vi "Scale Spectrum Information.vi"(8 "error in (no error)":errorcluster, 11 "Spectral Information (DBFS)":dbl[](array[numeric])) -> (0 "error out":errorcluster, 3 "Spectral Waveform":waveform(dbl))   [LabVIEW 2016]
uses:
  RTLSDR Control/RTLSDR Global Variables.vi
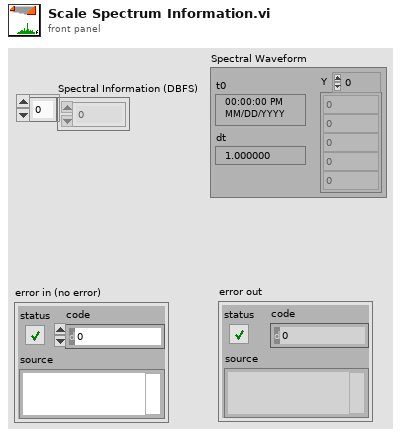
[diagram p1: front panel]
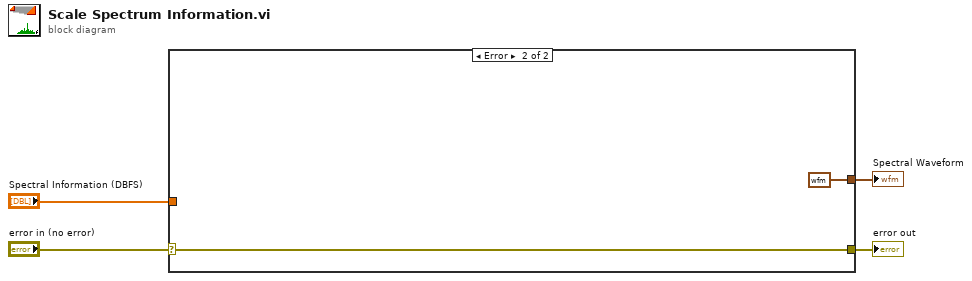
[diagram p0: block diagram]
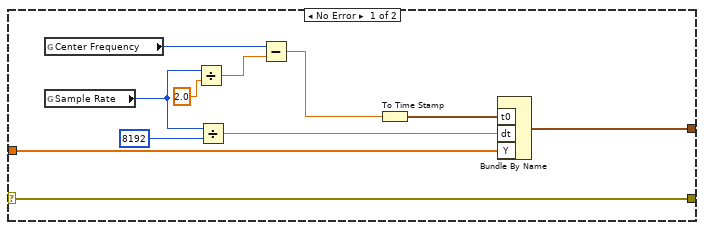
[diagram p2: hidden frame]
diagram:
  n1 = case shown="Error" "error in (no error)" {
    selector: "error in (no error)" -> [w10 w17]
    tunnel: "Spectral Information (DBFS)" -> [w6 _]
    tunnel: [w10 w17] -> w2
    tunnel: [w5 waveform(dbl) {"t0"=timestamp(0 s since 1904-01-01), "dt"=1.0, "Y"=[]}] -> w1
    frame No Error {
      n2 = global read "RTLSDR Global Variables.vi" "Center Frequency"() -> (w13:u32)
      n3 = global read "RTLSDR Global Variables.vi" "Sample Rate"() -> (w15:u32)
      n4 = Divide(x=w15, y=2.0) -> (x/y=w12:dbl)
      n5 = Divide(x=w15, y=u32 8192) -> (x/y=w7:dbl)
      n6 = Subtract(x=w13, y=w12) -> (x-y=w9:dbl)
      n7 = To Time Stamp(1:w9) -> (0:w8:timestamp)
      n8 = Bundle By Name("t0"=w8, "dt"=w7, "Y"=w6) -> (w5:waveform(dbl))  [unwired: 1 in]
    }
    frame Error {
    }
  }
  "error out" <- w2
  "Spectral Waveform" <- w1
